vi "ChannelMultiPlex.vi"(7 "start":i32, 9 "string":string, 10 "set following Variables":string[](array[string]), 11 "Numeric":i32) -> (2 "String":string, 3 "Array":string[](array[string]))   [LabVIEW 2011]
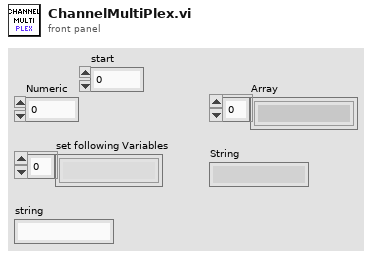
[diagram p1: front panel]
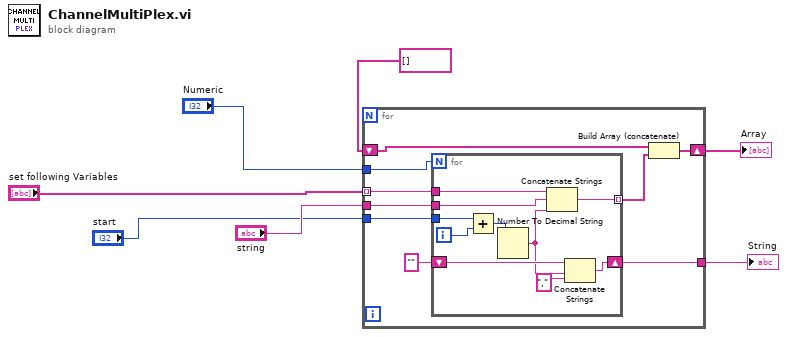
[diagram p0: block diagram]
diagram:
  n1 = for {
    tunnel: "Numeric" -> [w16]
    tunnel: [w14] -> w3
    tunnel: "set following Variables" -> [w13] mode=indexing
    shift-right: [w11] -> w5
    shift-left: string[] [] -> [w10]
    tunnel: "string" -> [w9]
    tunnel: "start" -> [w8]
    n2 = for {
      N: w16 -> [_]
      shift-right: [w25] -> w14
      shift-left: "" -> [w24]
      tunnel: w13 -> [w22]
      tunnel: [w21] -> w12 mode=indexing
      tunnel: w9 -> [w20]
      tunnel: w8 -> [w18]
      i -> [w19]
      n3 = Add(x=w18, y=w19) -> (x+y=w17:i32)
      n4 = Number To Decimal String(number=w17) -> (decimal integer string=w23:string)  [unwired: 1 in]
      n5 = Concatenate Strings(w22, w20, w23) -> (w21:string)
      n6 = Concatenate Strings(w24, w23, "," ("string")) -> (w25:string)
    }
    n7 = Build Array (concatenate)(w10, w12) -> (w11:string[])
  }
  "Array" <- w5
  "String" <- w3
